vi "FS Flip-Flop.vi"(8 "Button Value":bool, 10 "Current State":bool) -> (2 "result":bool)   [LabVIEW 2011, in "GripsMaster.lvclass"]
uses:
  GripsMaster.lvclass
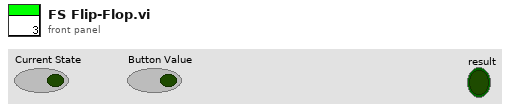
[diagram p1: front panel]
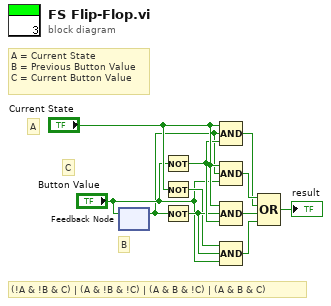
[diagram p0: block diagram]
diagram:
  # "A"
  # "C"
  # "B"
  # "A = Current State\nB = Previous Button Value\nC = Current Button Value"
  # "(!A & !B & C) | (A & !B & !C) | (A & B & !C) | (A & B & C)"
  n1 = feedback #1() -> (w1:bool)  [unwired: 1 in]
  n2 = feedback-in #1("Button Value") -> ()
  n3 = Not(x="Button Value") -> (.not. x?=w10:bool)
  n4 = Not(x="Current State") -> (.not. x?=w8:bool)
  n5 = Not(x=w1) -> (.not. x?=w9:bool)
  n6 = Compound Arithmetic op=AND("Current State", w1, w10) -> (w6:bool)
  n7 = Compound Arithmetic op=AND("Current State", w1, "Button Value") -> (w7:bool)
  n8 = Compound Arithmetic op=AND("Current State", w9, w10) -> (w5:bool)
  n9 = Compound Arithmetic op=AND(w8, w9, "Button Value") -> (w4:bool)
  n10 = Compound Arithmetic op=OR(w7, w6, w5, w4) -> (→"result":bool)
